vi "MT Calculate Power Adjustment and PAPR.vi"(5 "input complex waveform":T1 {"Y" format="%.3f"; "dt" format="%^.2e"; "t0" format="%.4f"}, 7 "waveform scaling factor":dbl=1.0, 11 "error in (no error)":errorcluster, 12 "reset?":bool=TRUE) -> (6 "Full Scale Adjustment (dB)":dbl caption="full scale adjustment (dB)", 8 "PAPR (dB)":dbl, 15 "error out":errorcluster)   [LabVIEW 2020, in "niDMT.lvlib"]
doc: "Returns the peak-to-average power ratio (PAPR) and the full-scale power adjustment."
uses:
  <vilib>/addons/Modulation/niDMT.lvlib
  <vilib>/addons/Modulation/Analog/controls/Complex Data Waveform.ctl
  <vilib>/addons/Modulation/niAMT.lvlib
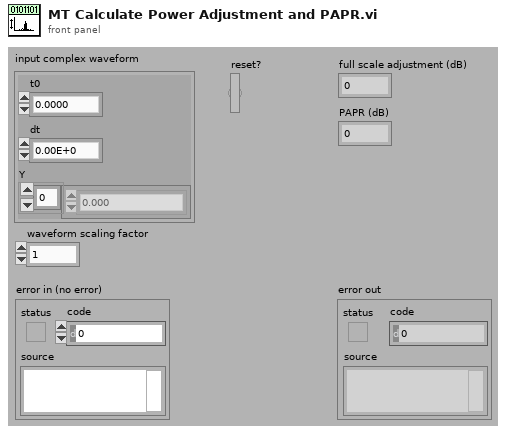
[diagram p1: front panel]
types:
  T1 = typedef "niAMT.lvlib/Complex Data Waveform.ctl" = cluster{"t0":dbl, "dt":dbl, "Y":cdb[]}
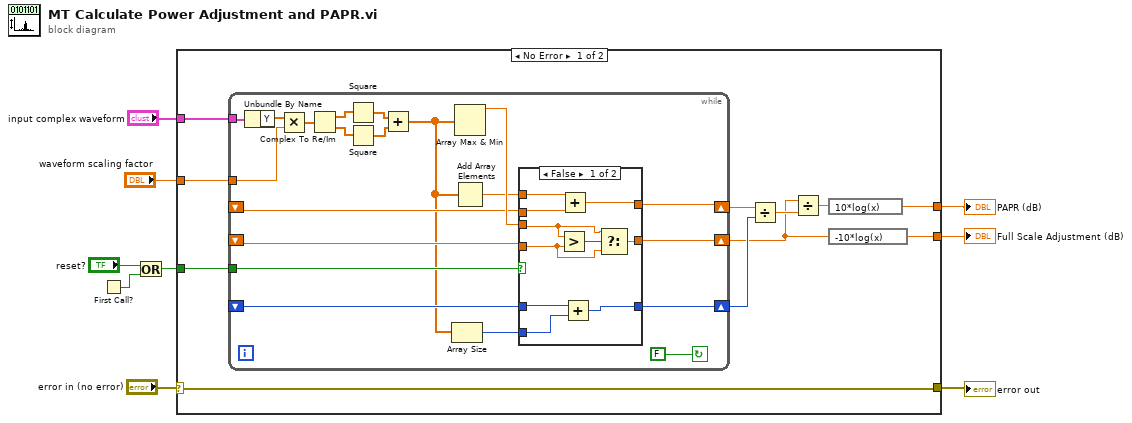
[diagram p0: block diagram]
diagram:
  n1 = First Call?() -> (First Call?: T/F=w7:bool)
  n2 = Or(x="reset?", y=w7) -> (x .or. y?=w6:bool)
  n3 = case shown="No Error" "error in (no error)" {
    selector: "error in (no error)" -> [w11 w54]
    tunnel: "input complex waveform" -> [w20 _]
    tunnel: w6 -> [w19 _]
    tunnel: [w15 _] -> w5
    tunnel: [w12 _] -> w4
    tunnel: [w11 w54] -> w3
    tunnel: "waveform scaling factor" -> [w10 _]
    frame No Error {
      n4 = while {
        tunnel: w20 -> [w40]
        shift-right: [w37] -> w13
        shift-left: _ -> [w39]
        tunnel: w19 -> [w36]
        shift-right: [w34] -> w14
        shift-left: _ -> [w33]
        shift-right: [w30] -> w18
        shift-left: _ -> [w32]
        tunnel: w10 -> [w27]
        stop <- FALSE continue-if-true
        n5 = Unbundle By Name(w40) -> ("Y"=w28:cdb[])
        n6 = Multiply(x=w28, y=w27) -> (x*y=w26:cdb[])
        n7 = Complex To Re/Im(x + iy=w26) -> (x=w25:dbl[], y=w24:dbl[])
        n8 = Square(x=w25) -> (x^2=w22:dbl[])
        n9 = Square(x=w24) -> (x^2=w23:dbl[])
        n10 = Add(x=w22, y=w23) -> (x+y=w21:dbl[])
        n11 = Array Size(array=w21) -> (size(s)=w31:i32)
        n12 = Array Max & Min(array=w21) -> (max value=w38:dbl)  [unwired: 3 out]
        n13 = Add Array Elements(numeric array=w21) -> (sum=w35:dbl)
        n14 = case shown="False" w36 {
          tunnel: w39 -> [w48 _]
          tunnel: w38 -> [w49 w51]
          tunnel: [w47 w51] -> w37
          tunnel: w35 -> [w46 w52]
          tunnel: [w44 w52] -> w34
          tunnel: w33 -> [w45 _]
          tunnel: w32 -> [w43 _]
          tunnel: w31 -> [w42 w53]
          tunnel: [w41 w53] -> w30
          frame False {
            n15 = Greater?(x=w49, y=w48) -> (0:w50:bool)
            n16 = Add(x=w46, y=w45) -> (x+y=w44:dbl)
            n17 = Add(x=w43, y=w42) -> (x+y=w41:i32)
            n18 = Select(t=w49, s=w50, f=w48) -> (s? t:f=w47:dbl)
          }
          frame True {
          }
        }
      }
      n19 = Divide(x=w14, y=w18) -> (x/y=w17:dbl)
      n20 = Divide(x=w13, y=w17) -> (x/y=w16:dbl)
      n21 = expression code="10*log(x)"(w16) -> (w15:dbl)
      n22 = expression code="-10*log(x)"(w13) -> (w12:dbl)
    }
    frame Error {
    }
  }
  "PAPR (dB)" <- w5
  "error out" <- w3
  "Full Scale Adjustment (dB)" <- w4
